vi "test_count4.vi"() -> ()   [LabVIEW 2013]
uses:
  <vilib>/fxp/LVFixedPointOverflowPolicyTypeDef.ctl
  <vilib>/fxp/LVFixedPointQuantizationPolicyTypeDef.ctl
  <vilib>/rvi/FXPMathLib/FxpConvert/subVIs/nifxpmath_Convert_SimConfig.ctl
  <vilib>/rvi/FXPMathLib/FxpConvert/simVIs/DllFxpConvertTemp_sub.vi
  <vilib>/rvi/FXPMathLib/FxpConvert/XNode/nifxpmath_Convert.xnode
panel:
  out "Waveform Graph 2":dbl[](graph)
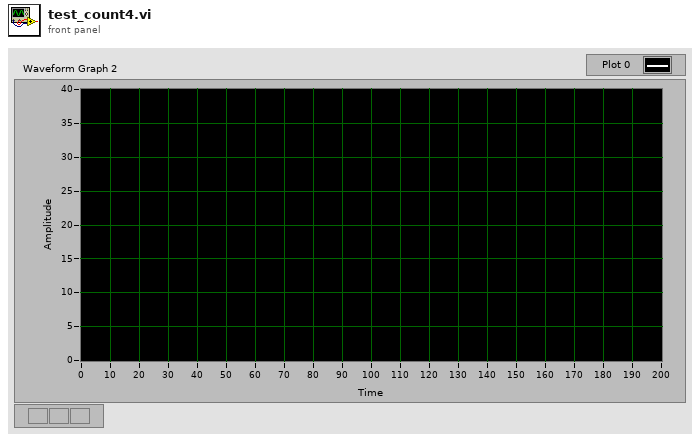
[diagram p1: front panel]
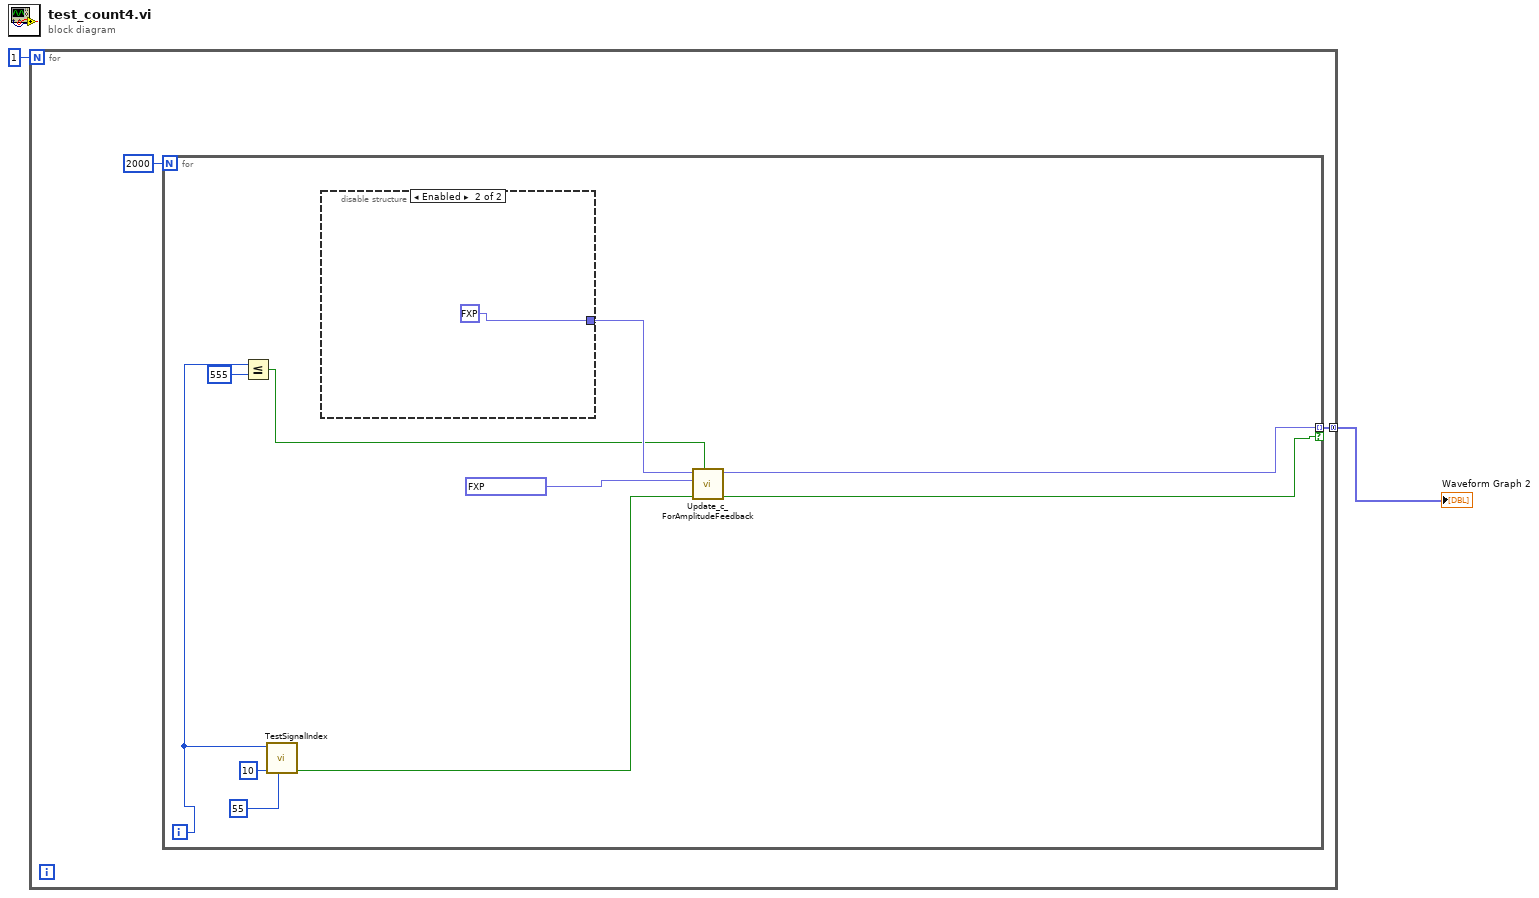
[diagram p0: block diagram]
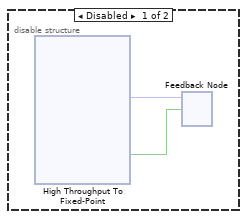
[diagram p2: hidden frame]
diagram:
  n1 = for {
    N: 1 -> [_]
    tunnel: [w3] -> w2 mode=concatenating
    n2 = for {
      N: 2000 -> [_]
      tunnel: [w7] -> w3 mode=indexing if=w6
      i -> [w12]
      n3 = Less Or Equal?(x=w12, y=555) -> (x <= y?=w5:bool)
      n4 = call "TestSignalIndex.vi"("initial delay"=55, "cycles per sample"=10, "index"=w12) -> ("valid out"=w9:bool)  [unwired: 7 in, 1 out]
      n5 = disable-structure shown="Enabled" {
        disable-tunnel: [_ fxp<+/-,32,21> 25.0 ("reset value")] -> w10
        frame Disabled {
          n6 = xnode "High Throughput To Fixed-Point"() -> ("x"=w17:fxp<+,16,14>, "y"=w16:fxp<+/-,32,21>, "input valid"=w18:bool, "output valid"=w15:bool)  [unwired: 1 in, 1 out]
          n7 = feedback #1() -> ()  [unwired: 2 in]
          n8 = feedback-in #1(w16, w15) -> ()
        }
        frame Enabled {
        }
      }
      n9 = call "Update_c_ForAmplitudeFeedback.vi"("Reset"=w5, "input valid"=w9, "delta_c"=fxp<+/-,32,21> 0.10009765625, "reset value"=w10) -> ("output valid"=w6:bool, "c out"=w7:fxp<+/-,32,21>)  [unwired: 6 in]
    }
  }
  "Waveform Graph 2" <- w2
